vi "DistToNearestStart.vi"(8 "Any Start":dbl, 9 "Z":dbl, 10 "X":dbl, 11 "All Lines 2":T1) -> (1 "Index":i32, 2 "Distance to nearest start":dbl, 3 "In range?":bool)   [LabVIEW 2014]
uses:
  Libraries/Map Data Folder/All-Lines.ctl
  Libraries/Map Data Folder/LineCluster.ctl
  Libraries/Map Data Folder/LineConnection.ctl
  Libraries/Map Data Folder/Map Data.lvlib
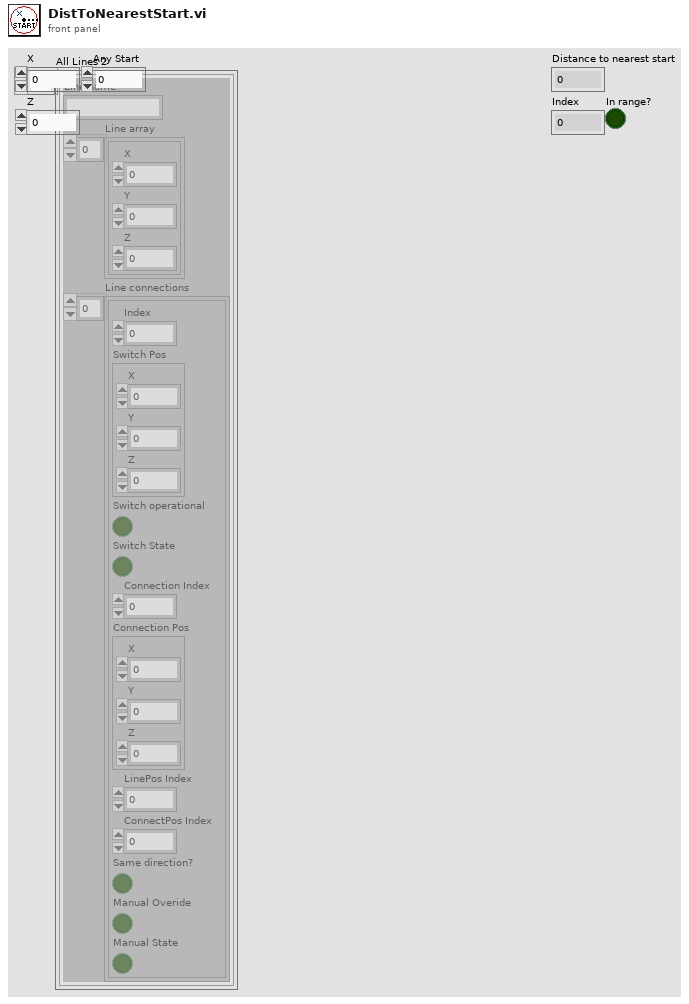
[diagram p1: front panel]
types:
  T1 = typedef "Map Data.lvlib/All-Lines.ctl" = T2[]
  T2 = typedef "Map Data.lvlib/LineCluster.ctl" = cluster{"Line name":string, "Line array":cluster{"X":dbl, "Y":dbl, "Z":dbl}[], "Line connections":T3[]}
  T3 = typedef "Map Data.lvlib/LineConnection.ctl" = cluster{"Index":i32, "Switch Pos":cluster{"X":dbl, "Y":dbl, "Z":dbl}, "Switch operational":bool, "Switch State":bool, "Connection Index":i32, "Connection Pos":cluster{"X":dbl, "Y":dbl, "Z":dbl}, "LinePos Index":i32, "ConnectPos Index":i32, "Same direction?":bool, "Manual Overide":bool, "Manual State":bool}
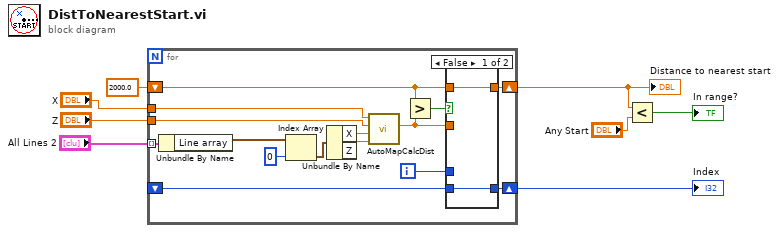
[diagram p0: block diagram]
diagram:
  n1 = for {
    tunnel: "All Lines 2" -> [w23] mode=indexing
    tunnel: "Z" -> [w22]
    tunnel: "X" -> [w21]
    shift-right: [w14] -> w3
    shift-left: 2000.0 ("Distance") -> [w13]
    shift-right: [w12] -> w4
    shift-left: _ -> [w10]
    i -> [w11]
    n2 = Unbundle By Name(w23) -> ("Line array"=w17:cluster{"X":dbl, "Y":dbl, "Z":dbl}[])
    n3 = Index Array(array=w17, index=0) -> (element=w18:cluster{"X":dbl, "Y":dbl, "Z":dbl})
    n4 = Unbundle By Name(w18) -> ("X"=w20:dbl, "Z"=w19:dbl)
    n5 = call "AutoMapCalcDist.vi"("Y2"=w19, "X2"=w20, "Y1"=w22, "X1"=w21) -> ("Distance"=w15:dbl)  [unwired: 7 in]
    n6 = Greater?(x=w13, y=w15) -> (0:w16:bool)
    n7 = case shown="False" w16 {
      tunnel: w15 -> [_ w27]
      tunnel: [w25 w27] -> w14
      tunnel: w13 -> [w25 _]
      tunnel: w10 -> [w24 _]
      tunnel: [w24 w26] -> w12
      tunnel: w11 -> [_ w26]
      frame False {
      }
      frame True {
      }
    }
  }
  "Distance to nearest start" <- w3
  "Index" <- w4
  n8 = Less?(x=w3, y="Any Start") -> (x < y?=→"In range?":bool)
